vi "WPI_AnalogChannelGetAveraging.vi"(8 "error in (no error)":errorcluster, 11 "AIDeviceRef":T1={"DevStatus"={"status"=FALSE, "code"=0, "source"=""}, "Analog Channel"=enum."AI 1"}) -> (0 "error out":errorcluster, 1 "OversampleBits":u8, 2 "AverageBits":u8, 3 "AIDeviceRef":T1={"DevStatus"={"status"=FALSE, "code"=0, "source"=""}, "Analog Channel"=enum."AI 1"})   [LabVIEW 2017]
doc: "Returns the number of bits the A/D converter uses to average the signal and the number of bits the converter uses to oversample the signal. Use the SetAveraging VI to set the number of bits to average and oversample.\n\nThis software is licensed. Open the labview\\readme\\WPI Robotics Library Open Source License.txt file for more information."
uses:
  <vilib>/Rock Robotics/WPI/AnalogChannel/WPI_AnalogChannelDevRef.ctl
  <vilib>/Rock Robotics/SystemInterfaces/AI/FPGA_AIChannel.ctl
  <vilib>/Rock Robotics/SystemInterfaces/System/FPGA_SystemGet.vi
  <vilib>/Rock Robotics/SystemInterfaces/AI/FPGA_AIOversampleBits.vi
  <vilib>/Rock Robotics/SystemInterfaces/AI/FPGA_AIERRInvalidAnalogChannel.vi
  <vilib>/Rock Robotics/SystemInterfaces/AI/FPGA_AIAverageBits.vi
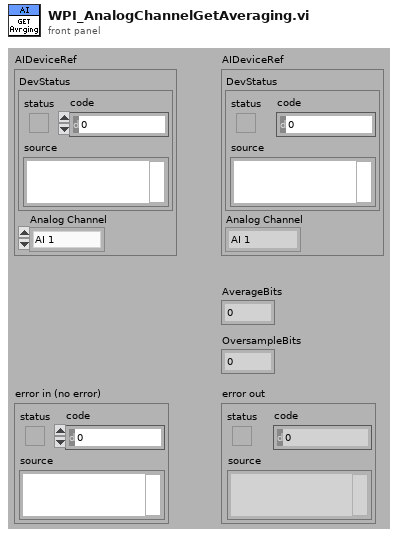
[diagram p1: front panel]
types:
  T1 = typedef "WPI_AnalogChannelDevRef.ctl" = cluster{"DevStatus":errorcluster, "Analog Channel":T2}
  T2 = typedef "FPGA_AIChannel.ctl" = enum8{"AI 0", "AI 1", "AI 2", "AI 3", "AI MXP 0", "AI MXP 1", "AI MXP 2", "AI MXP 3", "Invalid"}
  T3 = typedef "FPGA_AIDevRef.ctl" = cluster{"DevStatus":errorcluster}
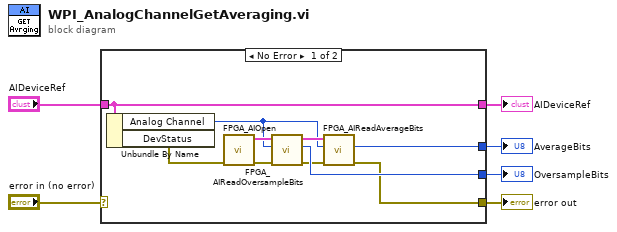
[diagram p0: block diagram]
diagram:
  n1 = case shown="No Error" "error in (no error)" {
    selector: "error in (no error)" -> [_ w17]
    tunnel: [w15 w18] -> w6
    tunnel: "AIDeviceRef" -> [w15 w18]
    tunnel: [w10 w17] -> w3
    tunnel: [w12 _] -> w2
    tunnel: [w14 _] -> w1
    frame No Error {
      n2 = Unbundle By Name(w15) -> ("Analog Channel"=w11:T2, "DevStatus"=w9:errorcluster)
      n3 = call <vilib>:"FPGA_AIOpen.vi"("error in (no error)"=w9) -> ("error out"=w8:errorcluster, "AI Reference out"=w16:T3)  [unwired: 2 in, 7 out]
      n4 = call <vilib>:"FPGA_AIReadOversampleBits.vi"("error in (no error)"=w8, "Channel"=w11, "AI Reference in"=w16) -> ("error out"=w7:errorcluster, "OversampleBits"=w12:u8, "AI Reference out"=w13:T3)  [unwired: 1 in, 5 out]
      n5 = call <vilib>:"FPGA_AIReadAverageBits.vi"("error in (no error)"=w7, "Channel"=w11, "AI Reference in"=w13) -> ("error out"=w10:errorcluster, "AverageBits"=w14:u8)  [unwired: 7 out]
    }
    frame Error {
    }
  }
  "AIDeviceRef" <- w6
  "OversampleBits" <- w2
  "error out" <- w3
  "AverageBits" <- w1
